vi "Create UI.vi"(8 "error in (no error)":errorcluster, 10 "instrument.PPMS2":refnum<class "instrument.PPMS2.lvclass">, 11 "Instrument.PPMS2 UI":refnum<class "Instrument.PPMS2 UI.lvclass">) -> (0 "error out":errorcluster, 3 "Instrument.PPMS2 UI out":refnum<class "Instrument.PPMS2 UI.lvclass">)   [LabVIEW 2016, in "Instrument.PPMS2 UI.lvclass"]
uses:
  Instrument.PPMS2 UI.lvclass
  C:/Program Files (x86)/National Instruments/LabVIEW 2016/vi.lib/JKI/JKI SMO/SMO/SMO.lvclass
  instrument.PPMS2/instrument.PPMS2.lvclass
  Instrument.PPMS2 UI.lvclass/Instrument.PPMS2 UI.ctl
  <vilib>/JKI/JKI SMO/SMO/SMO.lvclass
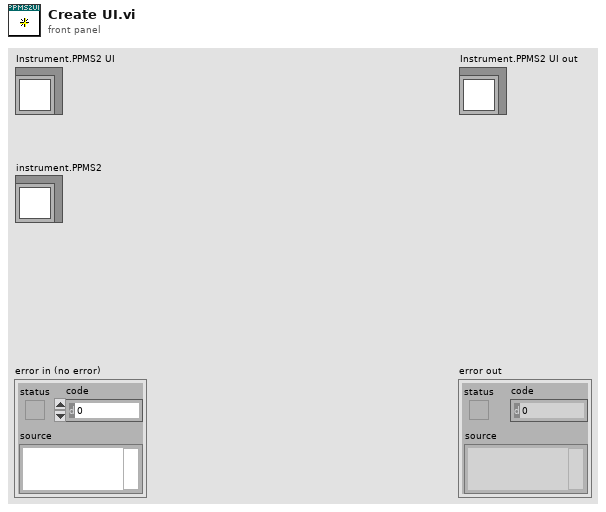
[diagram p1: front panel]
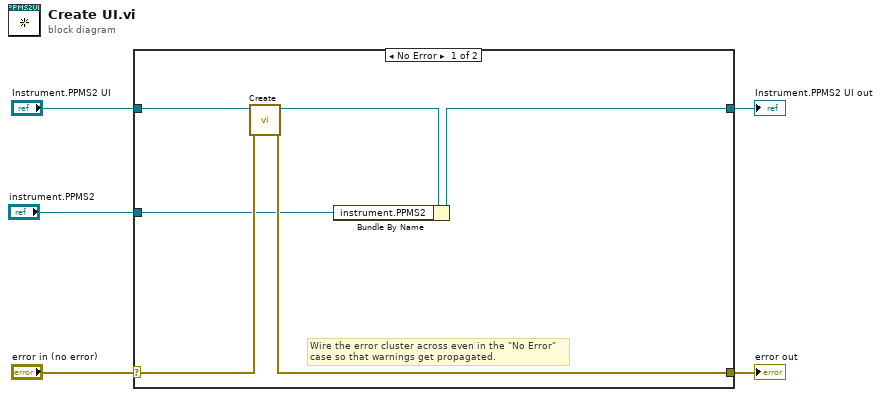
[diagram p0: block diagram]
diagram:
  n1 = case shown="No Error" "error in (no error)" {
    selector: "error in (no error)" -> [w8 w13]
    tunnel: [w7 w13] -> w4
    tunnel: [w11 w12] -> w2
    tunnel: "Instrument.PPMS2 UI" -> [w10 w12]
    tunnel: "instrument.PPMS2" -> [w6 _]
    frame No Error {
      # "Wire the error cluster across even in the \"No Error\"\ncase so that warnings get propagated."
      n2 = call <vilib>:"Create.vi"("error in (no error)"=w8, "SMO"=w10) -> ("error out"=w7:errorcluster, "SMO out"=w9:refnum<class "Instrument.PPMS2 UI.lvclass">)  [unwired: 7 in, 1 out]
      n3 = Bundle By Name(cluster=w9, "instrument.PPMS2"=w6) -> (w11:refnum<class "Instrument.PPMS2 UI.lvclass">)
    }
    frame Error {
    }
  }
  "error out" <- w4
  "Instrument.PPMS2 UI out" <- w2
